vi "Experiment-1.vi"() -> ()   [LabVIEW 2021]
uses:
  <vilib>/httpClient/LabVIEWHTTPClient.lvlib
panel:
  out "resulting string":string
  in  "Api key":string
  out "error out":errorcluster
  in  "error in (no error)":errorcluster
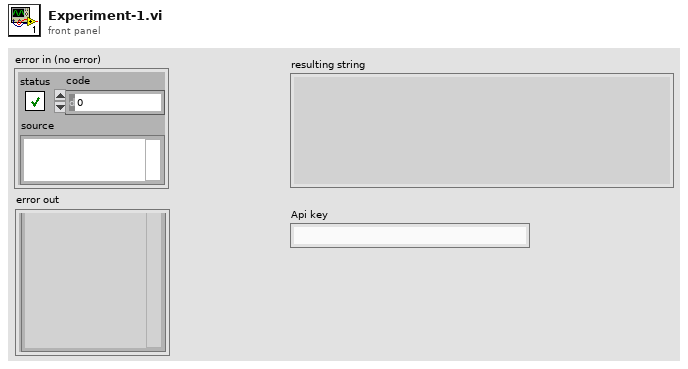
[diagram p1: front panel]
types:
  T1 = typedef "LabVIEWHTTPClient.lvlib/ClientHandle.ctl" = refnum<k1>
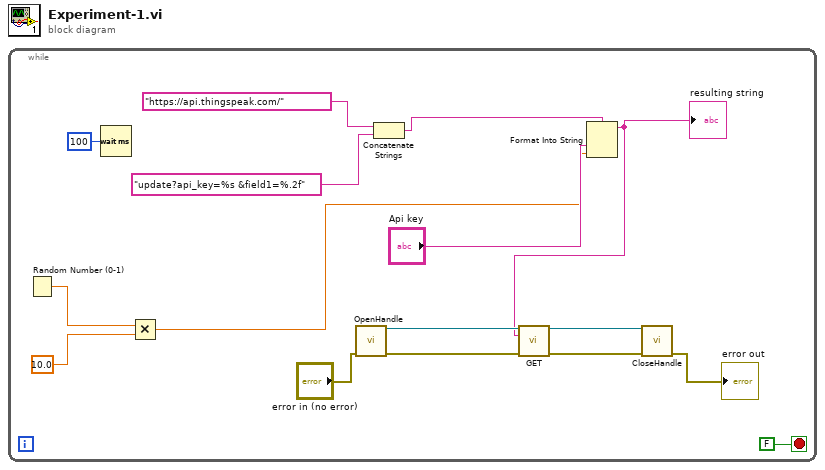
[diagram p0: block diagram]
diagram:
  n1 = while {
    stop <- FALSE stop-if-true
    n2 = Random Number (0-1)() -> (number: 0 to 1=w7:dbl)
    n3 = Wait (ms)(milliseconds to wait=u32 100) -> ()  [unwired: 1 out]
    n4 = Multiply(x=w7, y=10.0) -> (x*y=w2:dbl)
    n5 = call <vilib>:"OpenHandle.vi"("error in (no error)"="error in (no error)") -> ("client handle out"=w15:T1, "error out"=w14:errorcluster)  [unwired: 13 in]
    n6 = Concatenate Strings("https://api.thingspeak.com/" ("string"), "update?api_key=%s &field1=%.2f" ("string")) -> (w1:string)
    n7 = Format Into String(format string=w1, "Api key", w2) -> (resulting string=w4:string)  [unwired: 2 in, 1 out]
    "resulting string" <- w4
    n8 = call <vilib>:"GET.vi"("client handle"=w15, "url"=w4, "error in (no error)"=w14) -> ("client handle out"=w5:T1, "error out"=w13:errorcluster)  [unwired: 9 in, 2 out]
    n9 = call <vilib>:"CloseHandle.vi"("client handle"=w5, "error in (no error)"=w13) -> ("error out"=→"error out":errorcluster)  [unwired: 13 in]
  }
